vi "TestVI.vi"() -> ()   [LabVIEW 2023]
uses:
  MultiplyDLL.dll
panel:
  out "Product":dbl
  in  "B":dbl
  in  "A":dbl
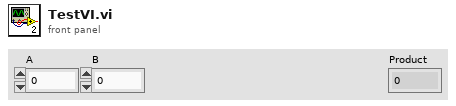
[diagram p1: front panel]
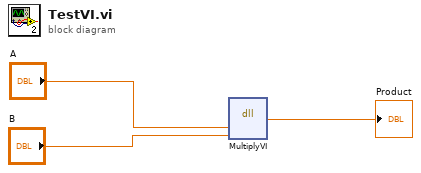
[diagram p0: block diagram]
diagram:
  n1 = dll-call lib="C:/Users/GKeerthi/Desktop/USER WORKFLOW/Build Output Deletion/DLL Files/MultiplyDLL.dll" fn="MultiplyVI"("A"="A", "B"="B") -> ("Product"=→"Product":dbl)  [unwired: 5 in, 2 out]
